vi "Restrict Motor by Encoder Value.vi"(5 "Disable Restrictor?":bool, 6 "Current Encoder Value":i32, 7 "Desired Power/Speed":i32, 9 "Lowest Position (degrees)":dbl, 10 "Highest Position  (degrees)":dbl) -> (2 "Output":i32)   [LabVIEW 2010, in "Tetrix.lvlib"]
uses:
  Tetrix.lvlib
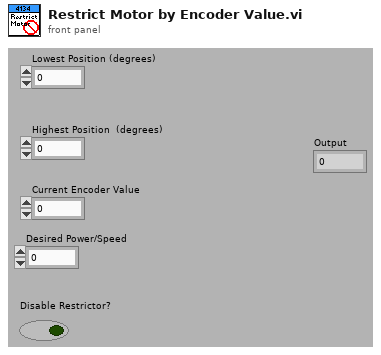
[diagram p1: front panel]
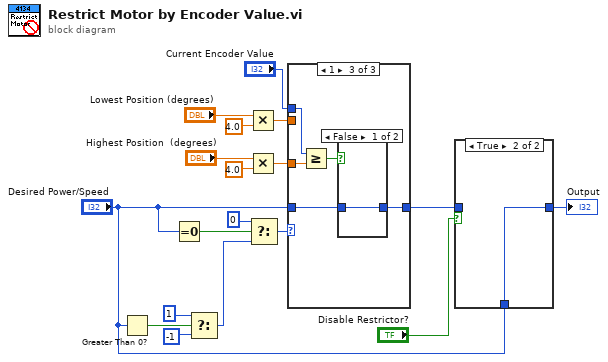
[diagram p0: block diagram]
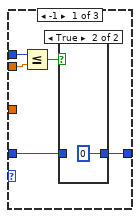
[diagram p3: hidden frame]
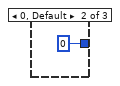
[diagram p5: hidden frame]
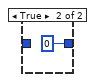
[diagram p6: hidden frame]
diagram:
  n1 = Greater Than 0?(x="Desired Power/Speed") -> (x > 0?=w12:bool)
  n2 = Equal To 0?(x="Desired Power/Speed") -> (x = 0?=w11:bool)
  n3 = Select(t=1, s=w12, f=-1) -> (s? t:f=w10:i32)
  n4 = Multiply(x="Lowest Position (degrees)", y=4.0) -> (x*y=w5:dbl)
  n5 = Multiply(x="Highest Position  (degrees)", y=4.0) -> (x*y=w6:dbl)
  n6 = Select(t=0, s=w11, f=w10) -> (s? t:f=w8:i32)
  n7 = case shown="1" w8 {
    tunnel: "Current Encoder Value" -> [w22 _ w31]
    tunnel: w6 -> [_ _ w30]
    tunnel: w5 -> [w21 _ _]
    tunnel: [w23 0 w27] -> w3
    tunnel: "Desired Power/Speed" -> [w19 _ w28]
    frame -1 {
      n8 = Less Or Equal?(x=w22, y=w21) -> (x <= y?=w20:bool)
      n9 = case shown="True" w20 {
        tunnel: [w24 0] -> w23
        tunnel: w19 -> [w24 _]
        frame False {
        }
        frame True {
        }
      }
    }
    frame 0, Default {
    }
    frame 1 {
      n10 = Greater Or Equal?(x=w31, y=w30) -> (x >= y?=w29:bool)
      n11 = case shown="False" w29 {
        tunnel: [w32 0] -> w27
        tunnel: w28 -> [w32 _]
        frame False {
        }
        frame True {
        }
      }
    }
  }
  n12 = case shown="True" "Disable Restrictor?" {
    tunnel: w3 -> [w34 _]
    tunnel: [w34 w35] -> w2
    tunnel: "Desired Power/Speed" -> [_ w35]
    frame False {
    }
    frame True {
    }
  }
  "Output" <- w2
